vi "Freefield Calibration.vi"(11 "IO Config File":path) -> ()   [LabVIEW 2020]
uses:
  epl-vi-lib/Utility VIs/Conversion VIs/Create Waveform Cluster (2D).vi
  Common VIs/Mic Sensitivity VIs/Cal Mic Sensitivity.vi
  epl-vi-lib/Connection VIs/Type Defs/CM-IO Type.ctl
  epl-vi-lib/Utility VIs/Math VIs/FFT x(t) to dB,Degrees (2D).vi
  Sub VIs/Tosca-Globals.vi
panel:
  in  "MicCalFile":path
  in  "Cal Mic Sens":dbl=-146.12351367888365 caption="Mic Sensitivity \n(dB V/SPL)" format="%.2f"
  in  "Meas Cal.M.Sen.":bool caption="Meas Ref.M.Sen."
  in  "UseMicCal":bool caption="Use mic calibration file?"
  in  "Smooth?":bool
  out "exit signal":bool
  in  "Exit":bool
  out "Abort":bool
  in  "Go":bool
  in  "Mic Gain (dB)":enum16{"0", "10", "20", "30", "40"}(ring)
  in  "Speaker":u16(ring)
  in  "Stimulus":T1={"Min Freq (Hz)"=1000.0, "Max Freq (Hz)"=50000.0, "Freq Step (Hz)"=50.0, "Waveform"=enum."Chirp", "Attenuation (dB)"=30.0, "Sample Rate (Hz)"=100000.0}
  out "Stimulus":cluster{i32, dbl, dbl[]}(graph)={0, 0.01, [-5.268198912753946, 0.15472436668775827, -4.936105719139354, 0.5336653168213406, -4.480102088018833, 1.008248465978206, -3.903407217524864, 1.5781086395910813, -3.213473335937858, 2.237701095068591, -2.422721892763888, 2.9756425911209785, -1.5491700358431084, 3.774205049267688, -0.6168718777938913, 4.609039499746465, 0.34390998389595134, 5.449215840646172, 1.2968922089759771, 6.25766663004243, 2.2004060816056343, 6.992118503588821, 3.008559346676577, 7.6065806282854345, 3.6729832875045987, 8.053433812076703, 4.145191339609901, 8.286124945969407, 4.379529507442163, 8.262418740636797, 4.336639279211482, 7.948093002561976, 3.9872822576766853, 7.320887614931534, 3.3162960756284035, 6.374435881980438, 2.3263695423908826, 5.121827480696606, 1.041250208545094, 3.598385074021946, -0.4920590232314779, 1.8631940827313715, -2.2025827080037574, -0.0010789574010842727, -3.996583101760993, -1.890495716744668, -5.761066652896276, -3.6845867196464788, -7.369807605524503, -5.253642640589705, -8.691888804601312, -6.4684195433316845, -9.602471024635907, -7.211803962263614, -9.995161830161347, -7.39162801642351, -9.794993105247707, -6.953467759606452, -8.970676902555233, -5.891950107327308, -7.544548237759553, -4.2588955339080545, -5.598484435293005, -2.1665998238617026, -3.2741767472418277, 0.2152325190333627, -0.7664729930576428, 2.669906820816478, 1.6908628776126302, 4.951744405784315, 3.846728261111973, 6.810894958294772, 5.460238707232009, 8.022997056956738, 6.331701759997024, 8.420539991290203, 6.333322125748589, 7.921776492633485, 5.435126476754877, 6.552446009009378, 3.7212991072610446, 4.455616406177521, 1.3925580613028812, 1.8858143442848072, -1.248492813884001, -0.8146341545862441, -3.8299221367236385, -3.2565671744760047, -5.958940837626473, -5.058652800945861, -7.28105198504492, -5.908941633849172, -7.541607328468995, -5.62378790744937, -6.63930777826804, -4.193115712222552, -4.660523620731457, -1.8013279613465976, -1.8847202037939093, 1.1842821697169106, 1.245000257577141, 4.260920175874573, 4.186397559561409, 6.87014224603152, 6.390599266533814, 8.499413795406833, 7.408308512375469, 8.78791295611658, 6.9897096713384315, 7.614861791824929, 5.155665436417732, 5.148471552216474, 2.2200736523520286, 1.8384841744623541, -1.2492218903049734, -1.6547038647773231, -4.531415502827719, -4.5875395794318745, -6.9012718876253345, -6.2956683656605055, -7.796639209855521, -6.356893664883222, -6.966612381173948, -4.714378044620799, -4.5603500004007325, -1.7230878322395136, -1.1252562365070526, 1.9034883988795923, 2.497808688702551, 5.246230005199975, 5.368578882073053, 7.4052822320392195, 6.689865512517134, 7.744589066651802, 6.037248961757495, 6.089605211597301, 3.5086613607099446, 2.814876655617855, -0.2603888568289086, -1.2188345294968457, -4.2380841595994045, -4.8785567401632814, -7.271376040922885, -7.077982229264194, -8.426667824565865, -7.1146351776726355, -7.296582121874083, -4.91986703319471, -4.169554633763585, -1.1293660738626015, 0.010491176358083346, 3.0712510234576733, 3.906409710496473, 6.300635894383965, 6.208952288616812, 7.437147684721125, 6.088644097766557, 6.027009247486187, 3.5212689620124986, 2.4930586247443416, -0.6457377872059515, -1.955346718576959, -4.940282413435899, -5.711814843262388, -7.768627179368542, -7.347657247363305, -8.010338407972391, -6.170204268617173, -5.483086055701031, -2.542906791186741, -1.0782044818065517, 2.187214902901886, 3.523630389730563, 6.167577492029727, 6.484585996632547, 7.768138306867664, 6.561596145324061, 6.278028385852266, 3.669742401891252, 2.267554919961306, -1.007135728576333, -2.5775918990285076, -5.454066706038607, -6.130112604803326, -7.670031202620425, -6.74903575803095, -6.575429386402428, -4.059732150963223, -2.566509572230266, 0.7941239410315287, 2.5800169685090917, 5.598533855668952, 6.469880615500485, 8.068262457243836, 7.213875021881164, 6.958454426976153, 4.387760938721065, 2.743633964491285, -0.6698285889953203, -2.5217172717892637, -5.436188670521526, -6.165478739199827, -7.440405214262041, -6.254625534425835, -5.563666428209676, -2.659960840977406, -0.7120378511037083, 2.7734736842514955, 4.561588179801471, 7.124215225716654, 7.371101211272586, 7.95487245705814, 6.091227796135417, 4.7104548555846355, 1.347640330347287, -0.8629413755604299, -4.2223764019046985, -5.6078946806208405, -7.403915239034967, -6.73948774271203, -6.280289141360928, -3.528182677804495, -1.4537578508184592, 2.151691445284337, 4.1924968824838205, 6.841173520638716, 7.163959080313049, 7.5742728334487355, 5.5198442779216625, 3.7800645182637878, 0.1883118086117216, -2.2308126826036725, -5.4902619476836, -6.626836451688596, -7.83306618297459, -6.508973280723542, -5.244810874956672, -1.8952004157835538, 0.606955058514041, 4.151452584017139, 5.7742997100602995, 7.483505877443789, 6.653165701726559, 5.707777580290299, 2.527839497455207, -0.0421815205393363, -3.785098469420861, -5.752805962190212, -7.801424804765037, -7.307010775975443, -6.564461661738033, -3.5029015548473668, -0.8999257692145889, 2.920120961873664, 5.031772146518852, 7.168610599551956, 6.7414300295566925, 5.961794404745086, 2.8441582282215334, 0.1338514074630595, -3.7271586992243555, -5.838810424147609, -7.843217323575976, -7.226392564538584, -6.172779494816889, -2.828986923398876, 0.05150957118887926, 3.898227328017297, 5.845970214987304, 7.487635305665838, 6.438529917848418, 4.922829795746704, 1.2708589242126918, -1.7202877354631272, -5.354532449742658, -6.832245596337666, -7.761997073930687, -5.961194594103097, -3.7683588570341477, 0.2570696544039717, 3.2603785999713053, 6.454848503138453, 7.173169225483685, 7.133981612463877, 4.444211132070024, 1.6238581609609706, -2.5228235439964717, -5.117128911369266, -7.3704847014121615, -6.861442815771931, -5.538160313137008, -1.8790767794661158, 1.3859193207825076, 5.2561678116596635, 6.937544346116766, 7.793213605118417, 5.796759070135655, 3.23732380929227, -1.0067099591150688, -4.056792333319176, -6.867337270546484, -6.926157676049868, -5.9480823057991135, -2.437329342060352, 0.9410718377756682, 5.003300952506423, 6.921678493302532, 7.870442069799751, 5.868846798920639, 3.15138312423561, -1.2262523447841607, -4.360520562115179, -7.039550600472367, -6.8254540193292925, -5.425058430665295, -1.5714782594174603, 1.9871958828743264, 5.860576249209403, 7.278450929372396, 7.435537663444447, 4.646116714214319, 1.3304854578842464, -3.142825361033163, -5.839027496935253, -7.53427953572099, -6.11784564901339, -3.587066735821253, 0.8669398004524809, 4.309913558664775, 7.230064109838996, 7.149607180067794, 5.619711454466257, 1.5585791296402056, -2.232363770655005, -6.085028073428171, -7.244657101692211, -6.844902187954905, -3.4915908929143473, 0.2346856222382626, 4.619909355449498, 6.728626808274241, 7.335598055639178, 4.738791826086019, 1.2546580511285206, -3.434169213629472, -6.294959617165018, -7.811616176072592, -6.006298392634771, -2.9243282833783684, 1.8263339552561098, 5.177408699038257, 7.38622013370554, 6.245568226203343, 3.5497386756087486, -1.18031166283291, -4.877402106803235, -7.624562302507592, -7.035732919059846, -4.691843955635915, -0.03916102015782511, 3.8698153755841718, 6.981994837389917, 6.781956858196558, 4.686291468984885, 0.09779697780872901, -3.9400841946319662, -7.263479231984435, -7.274681327948595, -5.282643435522408, -0.6918479981595833, 3.443619629756007, 6.865576168533289, 6.940338729493144, 4.932275215985484, 0.30236537946239417, -3.8570808228379367, -7.2075454948857605, -7.129379631590378, -4.91267407834013, -0.1361934643380461, 4.040346868467215, 7.216601071667613, 6.845491418147147, 4.32066005828306, -0.5985992815288892, -4.663224734534017, -7.443500502488409, -6.5381869393898775, -3.5301140426186146, 1.58258498272196, 5.4563056048440925, 7.687018074977699, 6.110612696861447, 2.5881403888345274, -2.6005475301936087, -6.04199444453435, -7.444864092474775, -4.992383767520014, -0.9077444233852652, 4.2342698830343375, 7.01788981780445, 7.387987352809551, 3.9967242643582868, -0.5092571824830199, -5.296631172179451, -7.070340682960906, -6.169613293871741, -1.8315435704147096, 2.8599819372393345, 6.919670453017385, 7.356344103481067, 5.080350143682289, -0.007085816050160075, -4.450717216127243, -7.306527333021936, -6.120738321455922, -2.5359997753017236, 2.8835512421863796, 6.487973207603957, 7.654891895746284, 4.7174230342389265, 0.1407496746273733, -4.979227860208258, -7.101779182600751, -6.264092701195794, -1.786090165267261, 3.0961184280731273, 7.05481129330459, 7.071743958604985, 4.167477970081142, -1.2938716831393164, -5.564824614463605, -7.554455584640754, -5.215261753753379, -0.7438685150851565, 4.63733729895058, 7.164584661085231, 6.552007283319558, 2.0676934427885048, -2.992900235336533, -7.04026615832861, -6.966438541255768, -3.7982072924186374, 1.8236464798201761, 5.960125196888981, 7.4140371618339165, 4.405395111049246, -0.5115316522716058, -5.715512079470977, -7.4486956056584654, -5.741118978332028, -0.5258040735298557, 4.421353351307599, 7.372267358024189, 5.741658380261856, 1.3522526983977523, -4.354569651532247, -7.288094350203355, -6.756543775969935, -2.0945874938808453, 3.1769460410787715, 7.042773160858427, 6.387686433421049, 2.4864168062370635, -3.39222429739403, -6.990987053298005, -7.159506000295234, -2.865999786873386, 2.533024409042783, 6.835427877890322, 6.6388697676783535, 2.9382852847908305, -3.017674445230749, -6.8505663481906875, -7.180577760890124, -2.9022704881692176, 2.5923158052172033, 6.925831567928834, 6.631494888469215, 2.7413917763985367, -3.2880358394581983, -6.953415262515216, -6.879496083870497, -2.2247260026423192, 3.3411092530878466, 7.273357193605295, 6.300652326252434, 1.852866676186904, -4.171172991169453, -7.186624607668294, -6.12902354187548, -0.7981910785525986, 4.652176578794313, 7.621054032499265, 5.397615158172362, 0.19659281853413826, -5.495756604067253, -7.219068212498481, -4.655291634956677, 1.3809179893349508, 6.2030315392201345, 7.485967672803411, 3.5807494650504568, -2.185222607280925, -6.832618016206194, -6.503842738222435, -2.1772446291201564, 4.089508811229626, 7.360481851909367, 6.2214480183612055, 0.6382302519063133, -4.886374544928762, -7.399486655729083, -4.4192288260547645, 1.2938205688827986, 6.6250384668429705, 7.171081058582159, 3.2897988000769116, -3.125494623688734, -6.911732715531365, -6.184970877676735, -0.6871977715566325, 5.026819820197494, 7.696981254517481, 4.695321242939161, -1.1624644088507237, -6.4866533422822386, -6.778679367154203, -2.537592715186285, 3.947887510720634, 7.320559752380773, 5.854035586827115, -0.13701600509322034, -5.637873695952034, -7.371155360792105, -3.359976713972514, 2.783840541352301, 7.262662307713002, 6.073547272708852, 0.7547535754815095, -5.477309421766594, -7.320704143407568, -4.076948523339965, 2.53079043139377, 6.879028855078228, 6.360929921143857, 0.6631898541259118, -5.2607397717088595, -7.593198682858205, -3.8811303142164526, 2.396208473538858, 7.097824106814894, 5.938217739780265, 0.438071984502258, -5.827153971326262, -7.3522200770230395, -3.583193416309296, 3.2037473262277665, 7.058746580825766, 5.5798006821120625, -0.7322933754485541, -6.2736137709411866, -7.282641773699037, -2.306637740796302, 4.079753813280838, 7.397921500073831, 4.346996330085451, -2.0204892667542436, -7.193316057455906, -6.356667865026697, -0.7775157490101203, 5.630597151405401, 7.024916096379502, 2.8515434851487265, -4.080310479287762, -7.455819131696737, -5.061730364173382, 1.7409273182319849, 6.716616268130217, 6.300852344279075, 0.23552513221494614, -5.812510898885256, -7.325656715369917, -2.416499935912286, 4.20595340691375, 7.503936045716031, 4.083013830130799, -2.576841185023463, -7.339719634050704, -5.523473316178671, 0.772215866457928, 6.689504274117393, 6.536788709293754, 0.9905473222769816, -5.6786287807560125, -7.072919350903344, -2.492595360069329, 4.610518393169291, 7.431512510272139, 4.008126798735533, -3.1803291782074385, -7.196110375032134, -4.972210543995063, 2.066365564079555, 7.08401321285749, 6.089340041167519, -0.5678580698696746, -6.342892846151588, -6.505666330592822, -0.35841099199108073, 5.985318681299599, 7.233767406971928, 1.7044686545440948, -5.014020375571299, -7.227374527708142, -2.3546475482644085, 4.592417575438715, 7.651973956236934, 3.443675179802632, -3.613300291172199, -7.397790861690395, -3.833752276459987, 3.238215867956934, 7.618538599317088, 4.637769723342312, -2.4043543328002115, -7.284534656947072, -4.8366282120338795, 2.124658179220868, 7.3833563562803715, 5.365786075012751, -1.5286689107614526, -7.101549908881539, -5.4522850675471135, 1.3553539065710465, 7.133510118326032, 5.727854230955125, -1.045904310760646, -6.989677300898881, -5.762167063662348, 0.9757983264882566, 6.985265407399975, 5.801261118091874, -0.9720815649171468, -7.0177242645731095, -5.809234307611887, 1.0039792584619325, 6.987323157037585, 5.6178467367115505, -1.3040770033795295, -7.18811195441027, -5.585445385131738, 1.4444012666063888, 7.123281681225336, 5.156842693841554, -2.026307886941771, -7.438605045603327, -5.032956777454607, 2.2836619932422635, 7.308768914377469, 4.350881349278516, -3.0988289576015937, -7.638971012985208, -4.059037989768774, 3.468094227327584, 7.38592769485375, 3.1079006313030444, -4.428347604106914, -7.588690184326886, -2.5693342094283067, 4.867003222988194, 7.12533243326591, 1.3551207959485267, -5.828292247585097, -7.029386568246263, -0.5255949468199037, 6.231850405988089, 6.252650257500143, -0.8903534092909058, -6.983645855777526, -5.691895386890709, 1.9717723677392618, 7.17394815534516, 4.5211080961372945, -3.4309862355822447, -7.450644081357213, -3.3973230722522314, 4.593486647599771, 7.1980976900131814, 1.8432618772903955, -5.809370417025735, -6.734255164992385, -0.21420006265580677, 6.731007664855428, 5.836152549849441, -1.5342489824366763, -7.304934828415726, -4.481433783316572, 3.370137858915535, 7.566115459500614, 2.901650517094279, -4.887209306299948, -7.0955274440845155, -0.7812482646532353, 6.373774279295743, 6.3445202532922576, -1.1890072905137836, -7.0452332506031565, -4.644004854227093, 3.541947226113793, 7.505870972955428, 2.8632692659772947, -5.211202610046928, -6.763474275312138, -0.24006791276950218, 6.890503265856279, 5.7417500312555525, -2.0055534494094984, -7.33737276359952, -3.4769048139735705, 4.604716101023941, 7.4088764134763965, 1.1882987138543064, -6.177258620815541, -5.986828798179214, 1.8531483144550864, 7.412557985728574, 4.13192051037388, -4.269852095724912, -7.1065896117768474, -1.1471485015074143, 6.512186887113054, 6.0211927787580235, -1.742035149083485, -7.375702831608887, -3.5159499563671814, 4.708021360701314, 7.21681111293023, 0.5253731768581403, -6.637719013896884, -5.472203173475872, 2.835983027958118, 7.4174703354896625, 2.674619443930915, -5.630851885441911, -6.575749936156022, 0.7909319027737999, 7.254060445787437, 4.1722214947775775, -4.2266678223662115, -7.330160415722715, -0.8252888610020537, 6.553516610912413, 5.418876561967503, -3.039107659742079, -7.480630271961402, -2.3188358948188736, 5.917107002494558, 6.084259196613284, -1.8109874183634276, -7.570939769222146, -3.2782185847135095, 5.113155616671117, 6.647524150125307, -1.0022706256615814, -7.349780692491279, -4.103765116699421, 4.629395585382437, 6.821925602548551, -0.2703686909901486, -7.292107730028471, -4.456559373064684, 4.1617649608314515, 7.049200144935046, 0.006196751679581222, -7.098805407130077, -4.731715940350453, 4.108203743544292, 7.013235776847501, 0.18415732468433557, -7.161584281268779, -4.591033378380794, 4.126429376001207, 7.0791935320889445, -0.08855841191627135, -7.135214960218198, -4.380778864995472, 4.553006058302461, 6.883801926906562, -0.4722410686728798, -7.332725197110119, -3.7437692063795662, 5.020095243935368, 6.71171645322024, -1.2985962708294916, -7.3622106844365875, -2.9800400656221955, 5.797291864656931, 6.158816331213153, -2.224937194593592, -7.452801625687471, -1.7381023125659305, 6.468183227507671, 5.449800363739938, -3.518314665836994, -7.161835192560194, -0.32239852080531084, 7.202750217326174, 4.182349566323476, -4.767726810954141, -6.645762480602695, 1.5338234973032108, 7.507271290643875, 2.5982763353206244, -6.100556932988706, -5.456445557052954, 3.415468302893055, 7.451267688369972, 0.4173032991800682, -6.974243481539636, -3.7796132692587077, 5.386226011801764, 6.521837729952901, -1.9391425150286377, -7.362910965180193, -1.3353108448939035, 6.824424409945794, 4.839741670112702, -4.4501670956283705, -6.67827190354844, 1.4212313376951484, 7.578245200127353, 2.137799252458786, -6.378976706181101, -4.977491033689597, 4.343053947340082, 6.968781033772617, -1.0532636822086119, -7.411520461688359, -2.0333166452809386, 6.533476295718684, 5.010056713625797, -4.394771409814594, -6.766415880577115, 1.490592054440969, 7.494701529741184, 1.584510348167756, -6.765875003379135, -4.453721736990209, 4.994836541078157, 6.380014914243036, -2.401240444331501, -7.468034788581953, -0.5629989372293054, 7.1014838380930385, 3.315790659763432, -5.984972866410088, -5.666022464878779, 3.6364444725496945, 6.979129540023752, -1.2187945093177486, -7.520358777665627, -1.7810364268856296, 6.768011954431605, 4.010298267709568, -5.43908213200435, -6.199981869315344, 3.1150740281930926, 7.045375361245859, -0.7962947891099998, -7.579039481647398, -1.9406637419191988, 6.663438416961239, 4.03793806415907, -5.577393444155123, -6.025675155876606, 3.3524447442922387, 6.972745469273113, -1.3615484849416026, -7.54283528682556, -1.2527409352797423, 7.027594011265683, 3.19902479985998, -6.164911155250056, -5.277446467439849, 4.483910180531211, 6.416848405230189, -2.6831794233556474, -7.371094897377518, 0.499084165392108, 7.363843648896164, 1.5304658331085685, -7.066614597985621, -3.4987236286655747, 6.012514092209379, 5.1208152069279045, -4.726888892085679, -6.339980396690471, 3.0280610687405236, 7.170596716367043, -1.2304909909162949, -7.405376290549076, -0.6024544481206826, 7.35908916056172, 2.4111240157942073, -6.661273890158799, -3.9276309786496135, 5.894783285661235, 5.359498291875047, -4.51463386051595, -6.269245318061246, 3.3201813644649016, 7.112088310331547, -1.5931758561482559, -7.31157058232791, 0.29015178357394994, 7.525804393455864, 1.460715386346605, -7.070159289724406, -2.6057496859138713, 6.7447285383244, 4.1321168455714385, -5.791908477270606, -4.946633731136702, 5.085574659161792, 6.099100503146692, -3.8367309287034863, -6.511230043001646, 2.924531690254378, 7.234452167248464, -1.57584944954651, -7.256400220654791, 0.6111775712249089, 7.5673672000412555, 0.6766388457356355, -7.268044098909321, -1.581971016051082, 7.22885018125015, 2.6970731358613524, -6.705531672246968, -3.4775791751495437, 6.398472526999905, 4.357344965207453, -5.753451680296769, -4.988423451542873, 5.262443474031636, 5.611980042519988, -4.587086048407322, -6.099349682927693, 3.986351788380044, 6.47678241551341, -3.3524691857209836, -6.844753534998459, 2.701548116804122, 7.006193817072543, -2.158652789159005, -7.287278289511652, 1.5019584261002876, 7.273655545638933, -1.0785289881197602, -7.500700710838877, 0.44759570639718305, 7.356818396055228, -0.1546115414097622, -7.55789351243099, -0.42850824296939377, 7.327754353537282, 0.5931062701371723, -7.523447506788368, -1.1123666046166072, 7.247374449411044, 1.159185250634697, -7.449901616205839, -1.601621464253939, 7.162883318038112, 1.5458102912476162, -7.376367409426471, -1.899450820362437, 7.107098850147537, 1.757433193486522, -7.328452716552958, -2.01011509029858, 7.098661566725419, 1.7971510342778039, -7.318639128727494, -1.9361943763208442, 7.142434753368789, 1.6648073852202323, -7.34656075225719, -1.6774727637188105, 7.229689176548243, 1.356767167247066, -7.3989251846347255, -1.2314375310024652, 7.337952987361621, 0.8673536650984877, -7.449104232450871, -0.5954147670466945, 7.430690391118509, 0.19198443473597804, -7.456709150233372, 0.22960505823745772, 7.457261141055401, -0.6679619947529072, -7.367759400114487, 1.233451712394734, 7.353906046052044, -1.6986391934598437, -7.116342517234951, 2.3897741199596085, 7.0467730089811695, -2.865978782777268, -6.628896894855508, 3.6481691703374213, 6.458171005742338, -4.107611838917467, -5.832329492619806, 4.926704590233439, 5.517187548057526, -5.326147906215478, -4.666950020678309, 6.1069514253257315, 4.175347079673148, -6.386398813093694, -3.1044632212483703, 7.034546908113638, 2.4269197401967855, -7.1199582301857305, -1.1698218514798955, 7.5289510859962805, 0.33166218770904743, -7.340876726227963, 1.036471629569474, 7.405929210953934, -1.9647783612357537, -6.875407655143098, 3.321820293891651, 6.5147262079528465, -4.220434647492109, -5.606263402883918, 5.399664376298967, 4.788269349404898, -6.106439584183898, -3.5270227628406747, 6.912582638807577, 2.2988016760946346, -7.246217682554448, -0.7954174368579265, 7.488884339759199, -0.696205046129878, -7.290279059088492, 2.2334387254592376, 6.8343818182803435, -3.7400204302108024, -6.022587668123615, 5.018196863144114, 4.848106750641775, -6.21925088014328, -3.478780042622402, 6.909607072125957, 1.7330235675491468, -7.480914404048713, -0.038068175043771364, 7.305467184454901, -1.9445184173264187, -7.021243676354168, 3.563101460592977, 5.863706867127409, -5.30019256611829, -4.709091588781449, 6.345380550046475, 2.716281625948426, -7.320885780942076, -0.9668260764181981, 7.349045869067955, -1.4098828132495977, -7.190992713412808, 3.195376456475068, 6.003887408701125, -5.2694991187727975, -4.67572044811709, 6.383900715158481, 2.485755581766223, -7.437021874893461, -0.4039453612946393, 7.283973152152595, -2.1241094084617758, -6.86536613448874, 4.142265082449705, 5.267387667723275, -6.0546740711016405, -3.4768414745568266, 7.064626570553517, 0.8872129934270778, -7.492742844867697, 1.5237077317000276, 6.864034305240107, -4.069849674206927, -5.488323475199265, 5.917276189626665, 3.3271072713237677, -7.197653739918008, -0.6908421330394027, 7.408965533095865, -2.025187400995709, -6.654673412230403, 4.612716930967556, 4.923420046978757, -6.392242558651788, -2.3878636424510074, 7.464374614775881, -0.4523468148347535, -7.107263295567351, 3.4119278069323333, 5.939846181696391, -5.663739538586874, -3.392413997277974, 7.23495552715241, 0.6557471437831315, -7.304522630414506, 2.695122036717736, 6.382835657680963, -5.113094128823615, -3.9498736502053196, 7.1336670310335295, 1.0930032543939112, -7.283955770137286, 2.37658627156351, 6.558282885289726, -5.049018440869571, -3.9488754943513236, 7.094554010811722, 1.0430377448665433, -7.318649642280466, 2.6642916523307383, 6.318810357585746, -5.3080138447779435, -3.5879739009830725, 7.304902607746897, 0.3105868538709081, -7.173051569327158, 3.3416830891067137, 5.800843030737964, -6.016406429204358, -2.6099276973106673, 7.437985995874678, -0.8968525383556791, -6.885618752640273, 4.533134164207345, 4.650562518060876, -6.770810693679945, -1.1458164399628608, 7.4553189773982576, -2.730496942614673, -5.968048217614874, 5.8160937074042485, 2.9176196034845336, -7.445941801944742, 1.0423410434064015, 6.761704783590702, -4.743195289910076, -4.343459165795438, 7.023307372493463, 0.29477931334295804, -7.30412375074616, 3.5280082327773696, 5.181401901962682, -6.6884161105715005, -1.5924568517472815, 7.301053959440679, -2.7713986307337652, -6.022404331580274, 6.005444758334429, 2.2165403487578135, -7.537010365189257, 1.8386853210947882, 6.1943032816067305, -5.8514795104740305, -2.991137106537487, 7.263806422763899, -1.6325202796756646, -6.647602385093664, 5.378321463779326, 3.009420866089287, -7.480091922619858, 1.2201284744109158, 6.467236472992606, -5.573021530453243, -3.238750984296706, 7.2626510188566336, -1.5472406664052007, -6.594104792863606, 5.526892945820245, 2.784430587244071, -7.477451135507415, 1.764318217766512, 6.193312632869459, -6.005931672119629, -2.385004143128125, 7.371659778348825, -2.5316991839326146, -5.851015812061519, 6.3777597681171905, 1.4848907989979554, -7.359259216876276, 3.383746118747219, 5.121608727602291, -6.8870327556741024, -0.3419386359895471, 7.122433920514759, -4.4142022511899, -4.030839287920141, 7.372883921446936, -1.0104055374690604, -6.453195007736038, 5.652879886395455, 2.7192391185379594, -7.414473281753894, 2.822296941112396, 5.587859533857973, -6.505030504056118, -0.6982352824551419, 7.3427523387040825, -4.375716527149005, -3.797948598192084, 7.403901054754664, -1.2467079300186006, -6.206915079577845, 6.219994502035965, 1.8812855918849696, -7.21356980341845, 3.7976300394487357, 4.768156324999836, -7.090085790515599, 0.9925870731971558, 6.620623009652825, -5.632886555814452, -2.037184094810564, 7.575272088198509, -3.5305398861309003, -4.476744989356374, 7.240062304831142, -0.8131785901705556, -6.383254786545178, 6.133344940765426, 1.7437276038378704, -7.2172822408269335, 4.1293447739209785, 4.184032033228714, -7.3455305194741225, 1.916008769188193, 5.880822464727152, -6.4792053898117565, -0.5970589961541429, 7.094065192957407, -5.187917469318833, -2.757153061838549, 7.396113436351452, -3.2854972826184152, -4.772191206712707, 7.240321435536306, -1.390723203248624, -6.116260305539997, 6.326525799026532, 0.7144743302731418, -7.149271494643727, 5.205911455748185, 2.4630009343718093, -7.461037971557037, 3.606922021743368, 4.167991786044972, -7.522291187896895, 2.091294519815033, 5.341956985845469, -6.98166385006456, 0.34819064048930004, 6.393126140437912, -6.360560920695885, -1.0955731847071088, 6.894051332299561, -5.31128869421998, -2.6148139354445465, 7.3176903788025305, -4.361174242102421, -3.7248310077122744, 7.262144728895676, -3.1334741187855837, -4.859125077652972, 7.232020831764564, -2.140904686041697, -5.561579941593053, 6.82217355800608, -0.9673442783996639, -6.307003775872721, 6.546333483332153, -0.10889010405423968, -6.649335246347242, 5.979804185381586, 0.8864521852085172, -7.087513362547955, 5.63525805083038, 1.5319780041595186, -7.17053248948962, 5.063007834971533, 2.3068148074477537, -7.409581717960173, 4.773225847086141, 2.7243202913087545, -7.339554481284766, 4.292218234970269, 3.2821597294340616, -7.4775878501999715, 4.130472963240131, 3.4859959755485463, -7.34012884129945, 3.793660480785639, 3.8458047177268, -7.44779328506394, 3.7963055342514855, 3.8544734570010535, -7.2970421897086934, 3.6265937914663144, 4.030757146799401, -7.411385874473106, 3.8058030970737717, 3.8522276659686474, -7.266874913102797, 3.806246091744156, 3.845238144087636, -7.389895721484403, 4.156818465616575, 3.4716794649841134, -7.235888055513042, 4.3135530577508225, 3.2664169443963242, -7.334222845400351, 4.811793140792276, 2.677396155101437, -7.119772494562921, 5.088949016008644, 2.251128502265069, -7.125606361762035, 5.683972067609279, 1.4257376939212443, -6.767245399921996, 6.012080776288262, 0.7650925939860065, -6.584130569254961, 6.6124766289028, -0.2957169615208086, -5.976538959742762, 6.875099697236678, -1.1671936162978764, -5.496883472445029, 7.337906727964457, -2.408418255116013, -4.539207794871777, 7.366080415601138, -3.394921421033718, -3.6811574912810503, 7.5005479621525435, -4.671748894791566, -2.3254495527029784, 7.090252623782934, -5.5733321909020255, -1.0925326475946708, 6.693542404862393, -6.62916932518457, 0.5878143467857476, 5.663594405868356, -7.1374088657337555, 2.034690139061274, 4.603217845992474, -7.626149145285267, 3.7780707617726983, 2.901644568189083, -7.382220854118887, 5.07131765514263, 1.2406343061383283, -6.969894247839067, 6.412049108213185, -0.9225769167783797, -5.713714378933332, 7.012943400617945, -2.8037500151205674, -4.272202999499362, 7.385704926316464, -4.871283360284997, -2.0677727581517775, 6.770669893032357, -6.257354174975097, 0.09388756265418087, 5.781674164983426, -7.408537555470525, 2.6607714855204208, 3.7854099254741804, -7.4632547405994085, 4.683998588640356, 1.5930505968580824, -6.972103264862576, 6.536723624612685, -1.23234583482215, -5.229875124110247, 7.241220620442128, -3.661784658335817, -3.044333861500277, 7.2701217022324265, -5.990169988709713, 0.010601058375152657, 5.83530790274474, -7.116313518357464, 2.8167495544053627, 3.7391157119716016, -7.432194251015661, 5.5774787332529066, 0.5736924884437822, -6.073795748434888, 7.056885013617561, -2.438869392571146, -3.859268385910383, 7.566825583605902, -5.397328715537654, -0.4315930839781542, 6.1855017982488025, -6.92993031010169, 2.8468492299796297, 3.7847227402904178, -7.291276430888082, 5.945921857850861, 0.1068066140819823, -5.5527130408794045, 7.361544561252553, -3.302854764414877, -2.713782604756743, 7.335432635857689, -6.272811942495798, 1.3077181212058375, 5.014901385184877, -7.204035331726785, 4.735019252899437, 1.6295085128878233, -6.420071110229997, 7.268196155607813, -2.645237058479404, -3.277007289895888, 7.304098779984496, -5.783672176568736, 0.6385538744153036, 5.406018520513537, -7.439435296959046, 4.835105570456163, 1.3124691389736631, -6.1836952557524585, 7.1011206267826745, -2.921447554485646, -3.042899043677755, 7.24305407094255, -6.51929379287791, 1.692989251741919, 4.288379249143579, -7.291352432686731, 5.493894263830298, -0.025555092643484087, -5.535061544588668, 7.51995648018632, -4.791451749474087, -1.0620161154010102, 6.013119972602393, -7.220192135671134, 3.5503435214875694, 2.1990106921883044, -6.884413948062836, 6.995941269328584, -3.1051878782565536, -3.0054815612269277, 6.788886138600794, -6.680281702352021, 1.9447621049865997, 3.6074132631046685, -7.465930601719045, 6.332135569697447, -1.902140956931149, -4.122664682247093, 7.0474697348311865, -6.182225617763155, 0.987450504016817, 4.307318187590881, -7.646712207746921, 5.94143549484391, -1.3449584990348453, -4.528858050616823, 7.10768785408077, -5.99784833818804, 0.7794946356385093, 4.42108425287248, -7.6375498884863315, 6.00203369972859, -1.4728095957933145, -4.296858306756864, 7.085913464756461, -6.203031539261085, 1.3332641517130461, 3.9667943343253453, -7.4504035593841635, 6.494700043196976, -2.2817930240452595, -3.393648821480432, 6.877443616438691, -6.698712303866614, 2.602286685842846, 2.8427906367481475, -6.896652714707194, 7.199266294726993, -3.7025533769798784, -1.7105730842705416, 6.17286490673505, -7.181228790818576, 4.411974362603514, 0.9111133126008619, -5.623338683285598, 7.655856904023626, -5.481327278263599, 0.8038624431073437, 4.539746330470848, -7.1028272275444815, 6.3144195946827955, -1.8034793181298114, -3.2483904158245327, 7.167792474870116, -7.016022070941451, 3.8957151466123237, 1.649844329305818, -5.7393904447400015, 7.4591403195870685, -4.814300882898643, 0.32087271721727045, 4.996538698910781, -7.2978703082598315, 6.711130057911584, -2.293421830197837, -2.5369531029189907, 6.693858365069438, -6.932942720410846, 4.400709250099052, 0.9019034938261111, -5.232011317335216, 7.728515412451815, -6.070763570839876, 2.185089788906171, 3.18497512246112, -6.485072255501045, 7.19882653714837, -4.060491616072468, -0.5652155517907376, 5.395678763147044, -7.445899300511558, 6.5232258101982925, -2.408875508855543, -2.4414291294209893, 6.3649006703149045, -7.177372308663665, 4.902131545975449, -0.27653122193389595, -4.440752073311796, 7.311123039342662, -7.0466075550413985, 3.748393713743228, 1.02259006190719, -5.4001375456527505, 7.232087194276419, -6.112028514800706, 2.095552535628311, 2.5832017567243586, -6.5448710518470605, 7.464729024695672, -5.721191514224175, 1.2430983905085926, 3.2196486214937696, -6.775658303016905, 6.966918995244128, -4.802347606366615, 0.056554421507401656, 4.166056710700625, -7.386812543479487, 7.064953041110443, -4.6480399347448955, -0.21922722215183704, 4.242266849206085, -7.224540473962878, 6.609292906955443, -4.069812515834563, -0.8140872189924999, 4.723683236382706, -7.581082223109541, 6.8943465836242614, -4.3427985603489425, -0.469462178283496, 4.364039955886553, -7.207588595028469, 6.660750006909448, -4.1956857038108595, -0.4647348677075911, 4.44014636783252, -7.378388720535737, 7.177959419666832, -4.910104882295666, 0.4978317402166672, 3.62107740135188, -6.742755836737935, 7.07716617306676, -5.133176897284266, 1.086507371731375, 3.1923705588144142, -6.5627663115627115, 7.601303168125049, -6.137992714004316, 2.6142504029866966, 1.7653083915202596, -5.3995497165282895, 7.265693650955702, -6.455623108589378, 3.6457992451237335, 0.6913697570813713, -4.540701657216105, 7.2941918125858995, -7.314651755628377, 5.443451838379087, -1.3929159782414229, -2.5253539878920357, 6.117504128857631, -7.103452803831995, 6.39270593621441, -2.9556306733107145, -0.7801763344754337, 5.025576518112384, -7.025156450689789, 7.653611065280121, -5.212964074433305, 2.0237385995352533, 2.514655796524144, -5.416700313688903, 7.437789037496328, -6.35146670518208, 4.137993946935715, 0.16865462993144453, -3.659568612997817, 6.927332596263885, -7.431917921081369, 6.612557912757376, -3.1852214785674757, -0.3530387039328028, 4.441250109869715, -6.515927788053014, 7.352441731410537, -5.44245088809795, 2.558701451575206, 1.6384412548980578, -4.909561009186394, 7.3571682926497814, -7.413776024981069, 5.903184192786667, -2.518499192366596, -1.185233442622366, 4.752469608436264, -6.805773431696228, 7.147484134991613, -5.476729606965427, 2.3647584242330506, 1.382949174298675, -4.8930453362168285, 7.065405272198576, -7.672280695037907, 6.153253878954251, -3.436302020902229, -0.4226128698540964, 3.7180407541296425, -6.480348766354185, 7.098179399949354, -6.474136454485295, 3.6426532951535378, -0.5222610682769486, -3.4399270792713987, 5.910215565733283, -7.777677166092991, 7.077816746051623, -5.594645433613681, 2.02223732342793, 1.0837745270214958, -4.775851271391948, 6.404313630179907, -7.457579802725881, 5.8363753036487855, -3.8172154357841546, -0.052325203982481555, 2.9882568383629526, -6.268888647828698, 7.2689154904253535, -7.686975230614976, 5.566010612822198, -3.228507996011473, -0.6363758037337859, 3.4308357711670774, -6.297269204086456, 6.975500085117721, -6.945698825894605, 4.69016617948911, -2.1460494539852277, -1.5417150317653114, 4.332408838518213, -6.8705231353602745, 7.557807273249924, -7.270805211030309, 5.188932445833566, -2.511446883467661, -0.8982089125610887, 3.8346601306280266, -6.163622442033808, 7.151556709854065, -6.798471493733942, 5.138369404823166, -2.4099118004303173, -0.6616980407435415, 3.8512448844467184, -6.108996369005021, 7.6340437522303395, -7.437771191224908, 6.421084881867248, -3.8022520400649107, 1.1474518489641143, 2.286587898785318, -4.578856429007744, 6.775340417057683, -6.971198708068286, 6.78505682712836, -4.52806759715431, 2.4105029477573092, 1.112481056787596, -3.4785918328681715, 6.351874561908106, -7.164147298952606, 7.959530077199515, -6.414124870856378, 5.034131310812939, -1.7691310832533527, -0.564047032536154, 3.9150164777187664, -5.453627230322887, 7.266337798570007, -6.788733230111092, 6.384115717306525, -3.8763587734437794, 1.8557407551913272, 1.5363012529118347, -3.6991024316185057, 6.363363399649101, -7.1876391635132855, 7.951182638424688, -6.761792831703346, 5.498582338374045, -2.750840348462315, 0.39029592983396066, 2.6262177119682213, -4.645865154596283, 6.519173521741171, -7.023548538732575, 6.946115491778043, -5.60984411368266, 3.75066742179143, -1.2162056218274702, -1.4178741499303906, 3.907530046503666, -6.01021423028047, 7.24503209243035, -7.85464809147212, 7.23111879607223, -6.165309620886804, 3.934962021362205, -1.8309267127370736, -1.063152858114128, 3.086975435248174, -5.475044135932798, 6.349672450482585, -7.3667386358493205, 6.54289328234181, -5.986677586550185, 3.6446452653741734, -2.020782000511449, -1.0466393445324098, 2.7829432157407172, -5.53525515857639, 6.405254099349906, -7.992905660269564, 7.397545241785114, -7.489087683170065, 5.4288857102026835, -4.306391039205678, 1.3481236453529608, 0.24456578057710482, -3.2173567916128936, 4.39135943096623, -6.528046221926871, 6.595337300485438, -7.3873494827883155, 6.10449021213772, -5.544248846760801, 3.1751534276434694, -1.722366457239506, -1.0843826809067085, 2.6978090978033453, -5.155494661255595, 6.197820180898688, -7.654662704144305, 7.643250594322533, -7.78725152771682, 6.633309993865312, -5.568244075889204, 3.580785530238637, -1.7622350662739208, -0.4752522546902493, 2.40866919524754, -4.236566233671953, 5.673014156944682, -6.559799236743594, 7.09665122804632, -6.786760078597537, 6.334110060962726, -4.9019201672270345, 3.6855866076011115, -1.4903134691589983, -0.035339203799032035, 2.469952832491278, -3.7647855622532918, 5.9041092243934035, -6.495071508526586, 7.935051201114419, -7.5369280417086815, 8.097232275909386, -6.673282892314059, 6.4236050163663325, -4.177563813006, 3.3983254502663707, -0.7079091459078674, -0.19700483897050605, 2.881752542441214, -3.4932084715589706, 5.758091883852156, -5.74259463340116, 7.297820081354564, -6.478547105850378, 7.209839208206819, -5.595422628049647, 5.571009356183328, -3.341000721607474, 2.778598391041956, -0.23425715478056194, -0.5597031380088721, 3.0644702027601585, -3.7670492512600147, 5.897820652995271, -6.236972852878438, 7.739157488663354, -7.543547188170974, 8.280732591336193, -7.504650496720316, 7.470644612084793, -6.192679953662271, 5.498650578141172, -3.897955422581154, 2.7405024745573643, -1.0580135805474216, -0.3234505793249378, 1.829941671555072, -3.1975876455216596, 4.295992277660061, -5.451988004088022, 5.969393781338585, -6.782887910930249, 6.625875179664726, -7.045910611220712, 6.206473719659867, -6.26091611224869, 4.809253398866243, -4.5920111312568, 2.659266657499252, -2.3094855058906987, 0.06450620946791424, 0.25801896386818457, -2.633684476159889, 2.772835758538232, -5.107976541452407, 4.932091456014839, -7.084143784987004, 6.501046364397496, -8.36806390979394, 7.333326855209402, -8.8591505270234, 7.377646525308829, -8.55078907516914, 6.672438728293716, -7.519903948601991, 5.331080627898659, -5.908734720274895, 3.5210350437129154, -3.902254766858653, 1.4403238815014463, -1.7045150121628725, -0.7056072539422032, 0.4833248828667927, -2.7242219290307896, 2.481253855807945, -4.451804397732298, 4.143744964845767, -5.7641366321582455, 5.367731427325334, -6.581846951995106, 6.095435319977688, -6.870905400088031, 6.312742146377243, -6.6391307889492, 6.044112974706465, -5.929784574261516, 5.345153089878375, -4.813378185576395, 4.29394027247128, -3.3787467178763175, 2.9820939551746326, -1.7242817751942958, 1.5063777026278393, 0.04999215840351548, -0.038592247188749935, 1.8490369770110349, -1.566180502704833, 3.5878677172503783, -3.001956329097272, 5.195002769454339, -4.286321452431311, 6.614378769667364, -5.3756797669265355, 7.80591442773415, -6.242369039243872, 8.74496988413574, -6.873618389291001, 9.420974896985152, -7.269806725470315, 9.835497254611841, -7.4422839283846205, 10.0, -7.410986098531348, 9.933499797995244, -7.202035688424697, 9.66029563928829, -6.84547280591735, 9.207892374793566, -6.373220050168512, 8.605201258042488, -5.8173432099340925, 7.881062366060826, -5.208636048832144, 7.063102929999032, -4.57553019921288, 6.176921747554907, -3.9433110346834335, 5.24557277245882, -3.3336068503970155, 4.289310003143563, -2.7641109338379293, 3.3255499629309044, -2.2484931464836535, 2.369006298505884, -1.7964583939632761, 1.4319522464482368, -1.4139128212047907, 0.5245699414692682, -1.1032038220195375, -0.3446500832260673, -0.8634062356042506, -1.1684910062417149, -0.6906338046178808, -1.940600436571016, -0.5783616248202543, -2.655112322318282, -0.517751584541918, -3.3063188039851843, -0.49797843339505965, -3.888407596704841, -0.5065589657816423, -4.395277932282514, -0.5296907331436173, -4.820446023285823, -0.55260960786453, -5.157049223297509, -0.5599773115618993, -5.39795628927423, -0.5363105805493877, -5.535989103840361, -0.46646284424612283, -5.564258565776937, -0.3361669974163001, -5.476613783627737, -0.1326439116728561]}
  in  "Averages":i32=128
  in  "Stop":bool
  in  "Show all":bool
  in  "Load":bool
  in  "Clear":bool
  out "Path":path
  out "Acquired":i32
  out "ASTF phase":cluster{"Frequency":dbl[], "Frequency":dbl[]}[](graph)
  out "ASTF mag":cluster{"Frequency":dbl[], "Frequency":dbl[]}[](graph)
  out "Mic phase graph":cluster{"offset":dbl, "dx":dbl, "Y":dbl[][]}(graph)
  out "Mic mag graph":cluster{"offset":dbl, "dx":dbl, "Y":dbl[][]}(graph)
  out "Mic signals":cluster{"offset":dbl, "dx":dbl, "Y":dbl[][]}(graph)
  # "Raw Data"
  # "Acoustic System Transfer Function"
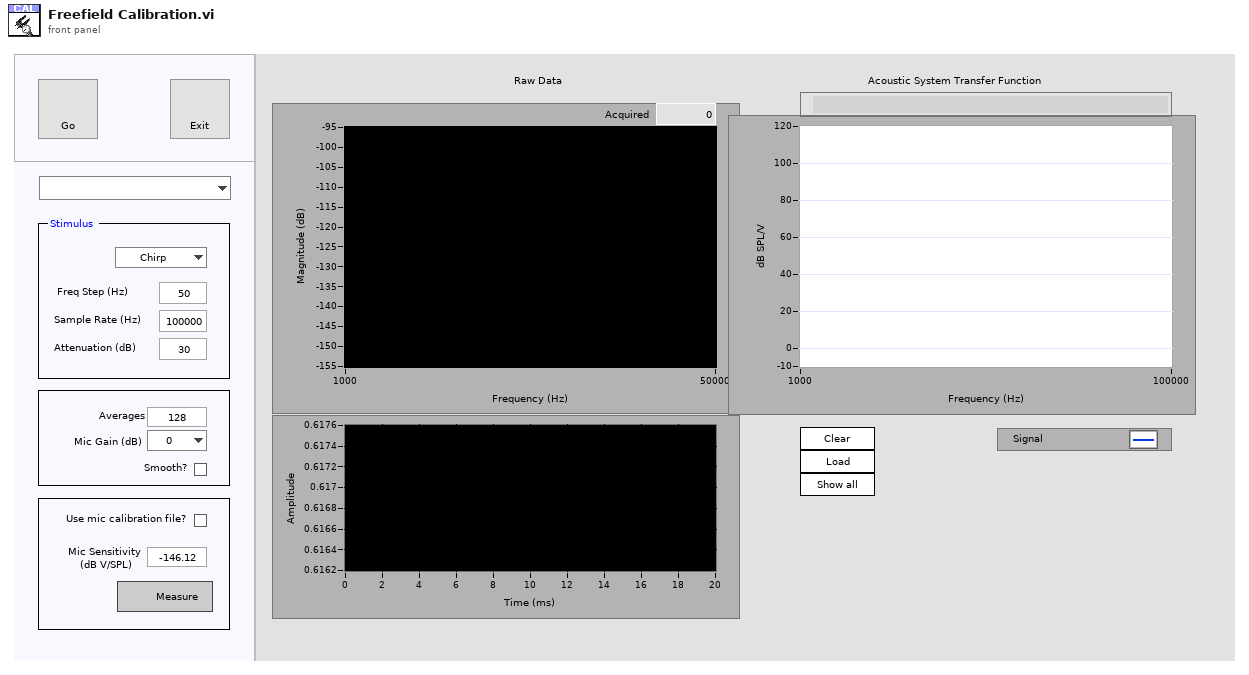
[diagram p1: front panel]
types:
  T1 = cluster{"Min Freq (Hz)":dbl, "Max Freq (Hz)":dbl, "Freq Step (Hz)":dbl, "Waveform":enum16{"Chirp"}, "Attenuation (dB)":dbl, "Sample Rate (Hz)":dbl}
  T2 = cluster{"Smooth?":bool, "Cal Mic Sens":dbl, "UseMicCal":bool, "MicCalFile ":path}
  T3 = typedef "CM-IO Type.ctl" = enum16{"Analog Outputs", "Analog Inputs", "Digital Outputs", "Digital Inputs"}
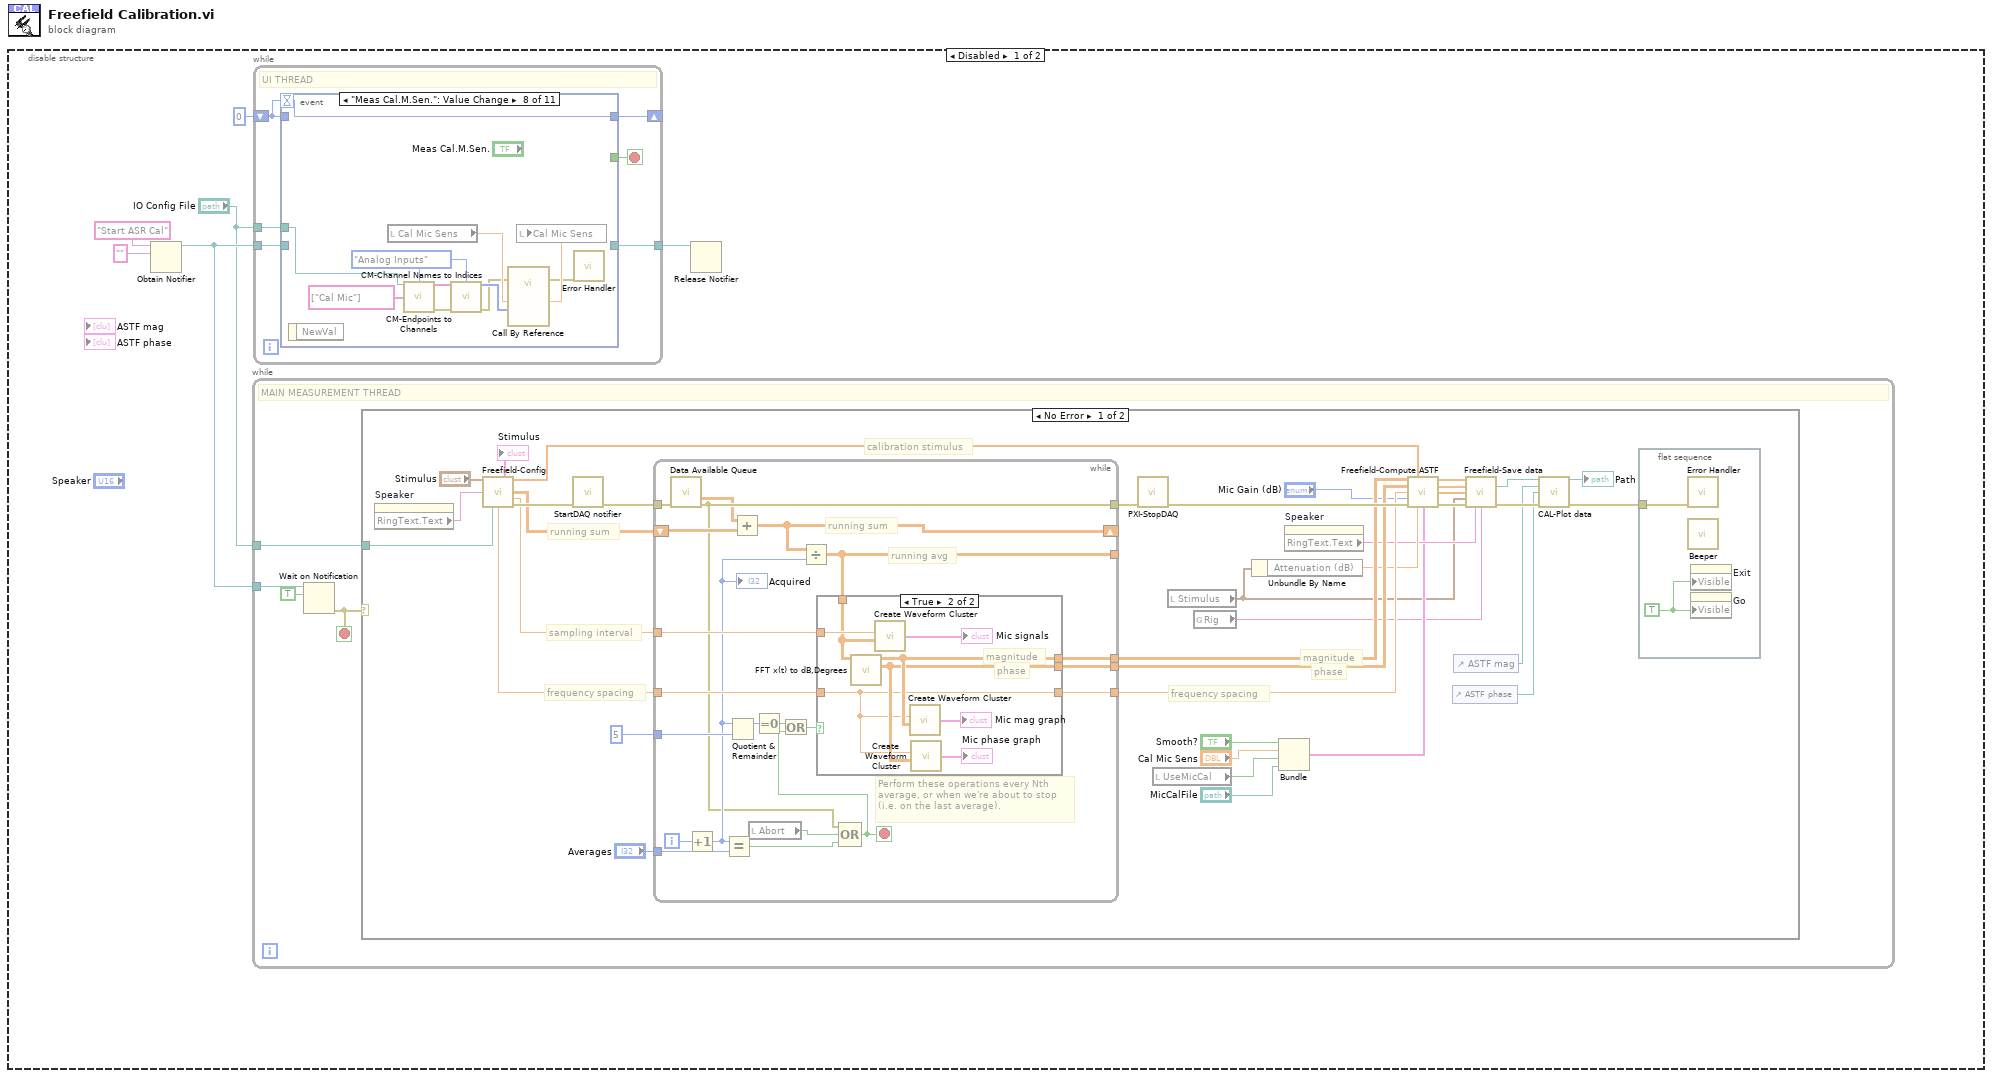
[diagram p0: block diagram]
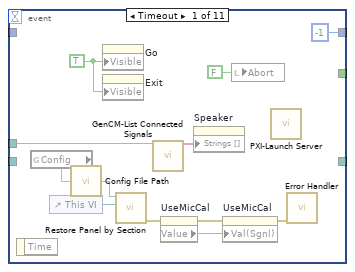
[diagram p4: hidden frame]
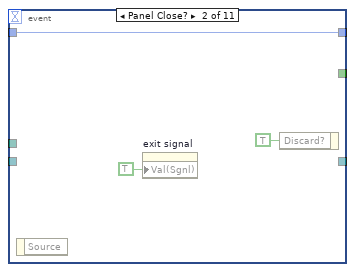
[diagram p5: hidden frame]
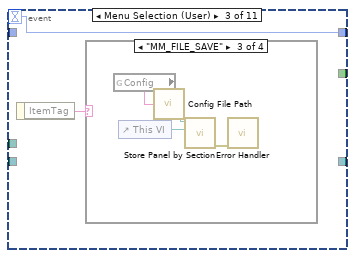
[diagram p6: hidden frame]
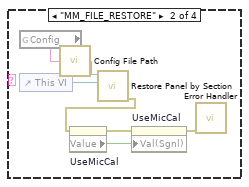
[diagram p8: hidden frame]
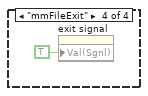
[diagram p9: hidden frame]
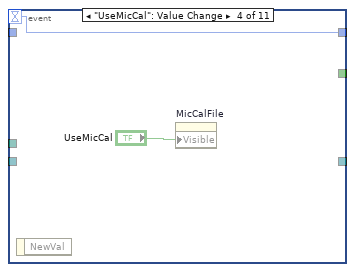
[diagram p10: hidden frame]
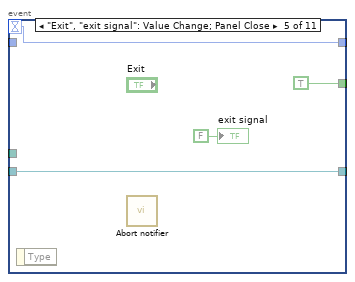
[diagram p11: hidden frame]
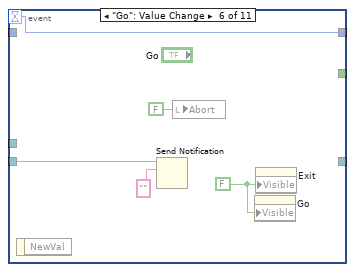
[diagram p12: hidden frame]
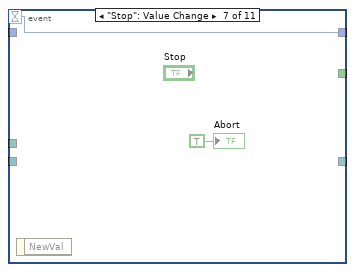
[diagram p13: hidden frame]
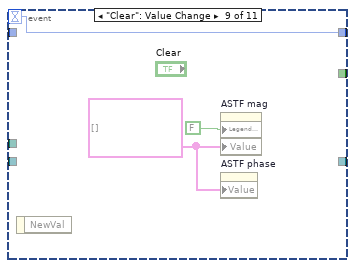
[diagram p14: hidden frame]
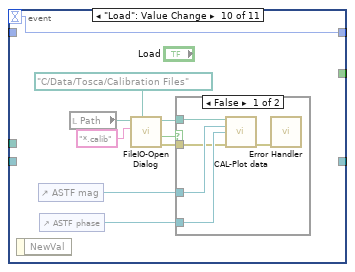
[diagram p15: hidden frame]
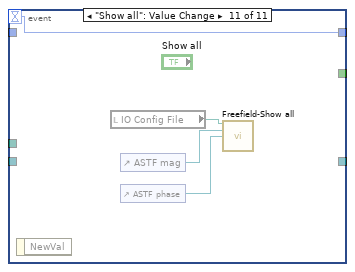
[diagram p17: hidden frame]
diagram:
  n1 = disable-structure shown="Disabled" {
    frame Disabled {
      n2 = Obtain Notifier(name (unnamed)="Start ASR Cal", notification data type="") -> (notifier out=w6:refnum<notifier>)  [unwired: 2 in, 2 out]
      n3 = while {
        tunnel: w6 -> [w9]
        tunnel: "IO Config File" -> [w7]
        stop <- w8 stop-if-true
        # "MAIN MEASUREMENT THREAD"
        n4 = Wait on Notification(notifier=w9, ignore previous (F)=TRUE) -> (error out=w8:errorcluster)  [unwired: 2 in, 3 out]
        n5 = case shown="No Error" w8 {
          tunnel: w7 -> [w13 _]
          frame No Error {
            # "phase"
            # "magnitude"
            # "frequency spacing"
            # "calibration stimulus"
            # "frequency spacing"
            # "sampling interval"
            # "running sum"
            n6 = property on="Speaker" class="Ring (strict)"() -> ("RingText.Text"=w12:string)  [unwired: 2 in, 2 out]
            n7 = call "Freefield-Config.vi"("Cal Stimulus"="Stimulus", "Speaker"=w12, "Path"=w13) -> ("Stimulus waveform"=→"Stimulus":cluster{i32, dbl, dbl[]}, "Stimulus"=w38:dbl[], "Mic Avg"=w46:dbl[][], "dt (ms)"=w44:dbl, "df (Hz)"=w45:dbl, "error out"=w47:errorcluster)  [unwired: 7 in]
            n8 = call "StartDAQ notifier.vi"("error in (no error)"=w47) -> ("error out"=w35:errorcluster)  [unwired: 6 in]
            n9 = while {
              tunnel: w35 -> [w70]
              tunnel: [w53] -> w34
              tunnel: "Averages" -> [w67]
              shift-right: [w65] -> _
              shift-left: w46 -> [w66]
              tunnel: [w51] -> _
              tunnel: 5 -> [w64]
              tunnel: w45 -> [w59]
              tunnel: [w58] -> w41
              tunnel: [w57] -> w40
              tunnel: w44 -> [w56]
              tunnel: [w55] -> w39
              i -> [w69]
              stop <- w60 stop-if-true
              # "Perform these operations every Nth\naverage, or when we're about to stop\n(i.e. on the last average)."
              # "running avg"
              # "running sum"
              n10 = call "Data Available Queue.vi"("error in (no error)"=w70) -> ("AI Waveforms"=w52:dbl[][], "error out"=w53:errorcluster)  [unwired: 10 in, 3 out]
              n11 = Increment(x=w69) -> (x+1=w54:i32)
              "Acquired" <- w54
              n12 = Equal?(x=w54, y=w67) -> (x = y?=w68:bool)
              n13 = Quotient & Remainder(x=w54, y=w64) -> (x-y*floor(x/y)=w63:i32)  [unwired: 1 out]
              n14 = Add(x=w52, y=w66) -> (x+y=w65:dbl[][])
              n15 = local read "Abort"() -> (w50:bool)
              n16 = Equal To 0?(x=w63) -> (x = 0?=w61:bool)
              n17 = Divide(x=w65, y=w54) -> (x/y=w51:dbl[][])
              n18 = Compound Arithmetic op=OR(w53, w50, w68) -> (w60:bool)
              n19 = Or(x=w61, y=w60) -> (x .or. y?=w62:bool)
              n20 = case shown="True" w62 {
                tunnel: w59 -> [_ w72]
                tunnel: [_ w76] -> w58
                tunnel: [_ w75] -> w57
                tunnel: w56 -> [_ w74]
                tunnel: [_ w72] -> w55
                tunnel: w51 -> [_ w71]
                frame False {
                }
                frame True {
                  # "phase"
                  # "magnitude"
                  n21 = call-poly "FFT x(t) to dB,Degrees.vi"("X(t)"=w71) -> ("+Freq Phase of FFT (degrees)"=w75:dbl[][], "+Freq. Mag of FFT (dB rms)"=w76:dbl[][])  [unwired: 9 in]
                  n22 = call-poly "Create Waveform Cluster.vi"("dx"=w74, "Array"=w71) -> ("waveform cluster"=→"Mic signals":cluster{"offset":dbl, "dx":dbl, "Y":dbl[][]})  [unwired: 3 in]
                  n23 = call-poly "Create Waveform Cluster.vi"("dx"=w72, "Array"=w76) -> ("waveform cluster"=→"Mic mag graph":cluster{"offset":dbl, "dx":dbl, "Y":dbl[][]})  [unwired: 3 in]
                  n24 = call-poly "Create Waveform Cluster.vi"("dx"=w72, "Array"=w75) -> ("waveform cluster"=→"Mic phase graph":cluster{"offset":dbl, "dx":dbl, "Y":dbl[][]})  [unwired: 3 in]
                }
              }
            }
            n25 = call "PXI-StopDAQ.vi"("error in (no error)"=w34) -> ("error out"=w43:errorcluster)  [unwired: 6 in]
            n26 = local read "UseMicCal"() -> (w17:bool)
            n27 = local read "Stimulus"() -> (w14:T1)
            n28 = global read "Tosca-Globals.vi" "Rig"() -> (w11:string)
            n29 = Unbundle By Name(w14) -> ("Attenuation (dB)"=w29:dbl)
            n30 = Bundle("Smooth?"="Smooth?", "Cal Mic Sens"="Cal Mic Sens", "UseMicCal"=w17, "MicCalFile"="MicCalFile") -> (w15:T2)  [unwired: 1 in]
            n31 = property on="Speaker" class="Ring (strict)"() -> ("RingText.Text"=w20:string)  [unwired: 2 in, 2 out]
            n32 = call "Freefield-Compute ASTF.vi"("Mag"=w41, "Stimulus"=w38, "Phase"=w40, "df (Hz)"=w39, "Mic Gain (dB)"="Mic Gain (dB)", "error in (no error)"=w43, "Attenuation (dB)"=w29, "Compute Options"=w15) -> ("ASTF Mag"=w30:dbl[], "ASTF Phase"=w25:dbl[], "Frequency"=w24:dbl[], "error out"=w31:errorcluster)  [unwired: 4 in]
            n33 = control-ref of="ASTF phase"() -> (w22:refnum<vi>)
            n34 = control-ref of="ASTF mag"() -> (w23:refnum<vi>)
            n35 = call "Freefield-Save data.vi"("Mag"=w30, "Phase"=w25, "Frequency"=w24, "Stimulus"=w14, "error in (no error)"=w31, "Speaker"=w20, "Rig"=w11) -> ("new file path"=w27:path, "error out"=w28:errorcluster)  [unwired: 7 in]
            n36 = call "CAL-Plot data.vi"("Path"=w27, "Mag graph"=w23, "Phase graph"=w22, "error in (no error)"=w28) -> ("Path (out)"=→"Path":path, "error out"=w42:errorcluster)  [unwired: 10 in]
            n37 = flat-sequence {
              tunnel: w42 -> [w49]
              frame #0 {
                w48 = TRUE
                n38 = call "Error Handler.vi"("error in (no error)"=w49) -> ()  [unwired: 13 in, 2 out]
                n39 = call "Beeper.vi"() -> ()  [unwired: 5 in, 1 out]
                n40 = property on="Exit" class="Bool"("Visible"=w48) -> ()  [unwired: 2 in, 2 out]
                n41 = property on="Go" class="Bool"("Visible"=w48) -> ()  [unwired: 2 in, 2 out]
              }
            }
          }
          frame Error {
          }
        }
      }
      n42 = while {
        tunnel: w6 -> [w83]
        tunnel: [w82] -> w3
        shift-right: [w81] -> _
        shift-left: 0 -> [w79]
        tunnel: "IO Config File" -> [w80]
        stop <- w84 stop-if-true
        # "UI THREAD"
        n43 = event shown="[7] \"Meas Cal.M.Sen.\": Value Change" {
          selector: _ -> [_ _ _ _ _ _ _ _ _ _ _]
          dyn-events: _ -> [_ _ _ _ _ _ _ _ _ _ _]
          timeout: w79 -> [_ _ w101 w115 w117 w121 w125 w135 w138 w147 w155]
          tunnel: [_ _ _ _ TRUE _ _ _ _ _ _] -> w84
          tunnel: w83 -> [_ _ _ _ w118 w124 _ _ _ _ _]
          tunnel: [_ _ _ _ w118 _ _ _ _ _ _] -> w82
          tunnel: [-1 w97 w101 w115 w117 w121 w125 w135 w138 w147 w155] -> w81
          tunnel: w80 -> [w86 _ _ _ _ _ _ w130 _ _ _]
          tunnel: w79 -> [_ w97 _ _ _ _ _ _ _ _ _]
          event Timeout {
            w95 = TRUE ("Visible")
            n44 = event-data() -> ()  [unwired: 1 in, 1 out]
            n45 = global read "Tosca-Globals.vi" "Config"() -> (w85:string)
            n46 = control-ref of="This VI"() -> (w91:refnum<vi>)
            n47 = call "Config File Path.vi"("AppName"=w85) -> ("Default config file name"=w90:path)
            n48 = property on="Go" class="Bool"("Visible"=w95) -> ()  [unwired: 2 in, 2 out]
            n49 = property on="Exit" class="Bool"("Visible"=w95) -> ()  [unwired: 2 in, 2 out]
            n50 = call "Restore Panel by Section.vi"("VI reference"=w91, "Path (dialog)"=w90) -> ("Error Out"=w92:errorcluster)  [unwired: 9 in]
            n51 = call "GenCM-List Connected Signals.vi"("Path"=w86) -> ("Analog Outputs"=w93:string[])  [unwired: 10 in, 4 out]
            n52 = property on="UseMicCal" class="Bool (strict)"(error in=w92) -> (error out=w89:errorcluster, "Value"=w87:bool)  [unwired: 1 in, 1 out]
            n53 = property on="Speaker" class="Ring (strict)"("Strings []"=w93) -> ()  [unwired: 2 in, 2 out]
            n54 = property on="UseMicCal" class="Bool (strict)"(error in=w89, "Val(Sgnl)"=w87) -> (error out=w88:errorcluster)  [unwired: 1 in, 1 out]
            n55 = local write "Abort"(FALSE ("Abort")) -> ()
            n56 = call "PXI-Launch Server.vi"() -> ()  [unwired: 10 in, 2 out]
            n57 = call "Error Handler.vi"("error in (no error)"=w88) -> ()  [unwired: 13 in, 2 out]
          }
          event Panel Close? {
            n58 = event-data() -> ()  [unwired: 1 in, 1 out]
            n59 = property on="exit signal" class="Bool (strict)"("Val(Sgnl)"=TRUE ("Value (Signaling)")) -> ()  [unwired: 2 in, 2 out]
            n60 = event-data("Discard?"=TRUE) -> ()  [unwired: 1 in, 1 out]
          }
          event Menu Selection (User) {
            n61 = event-data() -> ("ItemTag"=w100:string)  [unwired: 1 in]
            n62 = case shown="\"MM_FILE_SAVE\"" w100 {
              frame "False", Default {
              }
              frame "MM_FILE_RESTORE" {
                n63 = global read "Tosca-Globals.vi" "Config"() -> (w103:string)
                n64 = control-ref of="This VI"() -> (w108:refnum<vi>)
                n65 = call "Config File Path.vi"("AppName"=w103) -> ("Default config file name"=w102:path)
                n66 = call "Restore Panel by Section.vi"("VI reference"=w108, "Path (dialog)"=w102) -> ("Error Out"=w104:errorcluster)  [unwired: 9 in]
                n67 = property on="UseMicCal" class="Bool (strict)"(error in=w104) -> (error out=w105:errorcluster, "Value"=w107:bool)  [unwired: 1 in, 1 out]
                n68 = property on="UseMicCal" class="Bool (strict)"(error in=w105, "Val(Sgnl)"=w107) -> (error out=w106:errorcluster)  [unwired: 1 in, 1 out]
                n69 = call "Error Handler.vi"("error in (no error)"=w106) -> ()  [unwired: 13 in, 2 out]
              }
              frame "MM_FILE_SAVE" {
                n70 = global read "Tosca-Globals.vi" "Config"() -> (w110:string)
                n71 = control-ref of="This VI"() -> (w111:refnum<vi>)
                n72 = call "Config File Path.vi"("AppName"=w110) -> ("Default config file name"=w109:path)
                n73 = call "Store Panel by Section.vi"("VI reference"=w111, "Path (dialog)"=w109) -> ("Error Out"=w112:errorcluster)  [unwired: 9 in]
                n74 = call "Error Handler.vi"("error in (no error)"=w112) -> ()  [unwired: 13 in, 2 out]
              }
              frame "mmFileExit" {
                n75 = property on="exit signal" class="Bool (strict)"("Val(Sgnl)"=TRUE ("Value (Signaling)")) -> ()  [unwired: 2 in, 2 out]
              }
            }
          }
          event "UseMicCal": Value Change {
            n76 = event-data() -> ()  [unwired: 1 in, 1 out]
            n77 = property on="MicCalFile" class="Path"("Visible"="UseMicCal") -> ()  [unwired: 2 in, 2 out]
          }
          event "Exit", "exit signal": Value Change; Panel Close {
            n78 = event-data() -> ()  [unwired: 1 in, 1 out]
            n79 = call "Abort notifier.vi"() -> ()  [unwired: 6 in, 2 out]
            "exit signal" <- FALSE ("exit signal")
          }
          event "Go": Value Change {
            w120 = FALSE
            n80 = event-data() -> ()  [unwired: 1 in, 1 out]
            n81 = Send Notification(notification="", notifier=w124) -> ()  [unwired: 1 in, 2 out]
            n82 = local write "Abort"(FALSE ("Abort")) -> ()
            n83 = property on="Go" class="Bool"("Visible"=w120) -> ()  [unwired: 2 in, 2 out]
            n84 = property on="Exit" class="Bool"("Visible"=w120) -> ()  [unwired: 2 in, 2 out]
          }
          event "Stop": Value Change {
            n85 = event-data() -> ()  [unwired: 1 in, 1 out]
            "Abort" <- TRUE ("Abort")
          }
          event "Meas Cal.M.Sen.": Value Change {
            w132 = CM-IO_Type."Analog Inputs" ("IO Type")
            n86 = event-data() -> ()  [unwired: 1 in, 1 out]
            n87 = local read "Cal Mic Sens"() -> (w136:dbl)
            n88 = call "CM-Endpoints to Channels.vi"("Path"=w130, "IO Type"=w132, "Requested Endpoints"=string[] ["Cal Mic"] ("Inputs")) -> ("IO Channels"=w131:string[], "error out"=w133:errorcluster)  [unwired: 11 in]
            n89 = call "CM-Channel Names to Indices.vi"("IO Channels"=w131, "IO Type"=w132, "error in (no error)"=w133) -> ("Indices"=w129:i32[], "error out"=w128:errorcluster)  [unwired: 11 in]
            n90 = call-by-ref "?"(error in=w128, "AI Channels"=w129, "Mic Sens (dB V/SPL) in"=w136) -> (error out=w127:errorcluster, "Mic Sens (dB V/SPL)"=w137:dbl)  [unwired: 10 in, 1 out]
            n91 = local write "Cal Mic Sens"(w137) -> ()
            n92 = call "Error Handler.vi"("error in (no error)"=w127) -> ()  [unwired: 13 in, 2 out]
          }
          event "Clear": Value Change {
            w139 = cluster{"Frequency":dbl[], "Frequency":dbl[]}[] [] ("ASTF mag")
            n93 = event-data() -> ()  [unwired: 1 in, 1 out]
            n94 = property on="ASTF mag" class="XYGraph (strict)"("Legend Visible"=FALSE ("Legend:Visible"), "Value"=w139) -> ()  [unwired: 2 in, 2 out]
            n95 = property on="ASTF phase" class="XYGraph (strict)"("Value"=w139) -> ()  [unwired: 2 in, 2 out]
          }
          event "Load": Value Change {
            n96 = event-data() -> ()  [unwired: 1 in, 1 out]
            n97 = control-ref of="ASTF mag"() -> (w149:refnum<vi>)
            n98 = control-ref of="ASTF phase"() -> (w148:refnum<vi>)
            n99 = local read "Path"() -> (w143:path)
            n100 = call "FileIO-Open Dialog.vi"("Default Folder"=path "C:/Data/Tosca/Calibration Files", "pattern (all files)"="*.calib", "Start path"=w143) -> ("error out"=w146:errorcluster, "cancelled"=w145:bool, "selected path"=w144:path)  [unwired: 6 in]
            n101 = case shown="False" w145 {
              tunnel: w144 -> [w154 _]
              tunnel: w149 -> [w153 _]
              tunnel: w148 -> [w152 _]
              tunnel: w146 -> [w150 _]
              frame False {
                n102 = call "CAL-Plot data.vi"("Path"=w154, "Mag graph"=w153, "Phase graph"=w152, "error in (no error)"=w150) -> ("error out"=w151:errorcluster)  [unwired: 10 in, 1 out]
                n103 = call "Error Handler.vi"("error in (no error)"=w151) -> ()  [unwired: 13 in, 2 out]
              }
              frame True {
              }
            }
          }
          event "Show all": Value Change {
            n104 = event-data() -> ()  [unwired: 1 in, 1 out]
            n105 = local read "IO Config File"() -> (w156:path)
            n106 = control-ref of="ASTF mag"() -> (w158:refnum<vi>)
            n107 = control-ref of="ASTF phase"() -> (w157:refnum<vi>)
            n108 = call "Freefield-Show all.vi"("Path"=w156, "Mag graph"=w158, "Phase graph"=w157) -> ()  [unwired: 12 in, 1 out]
          }
        }
      }
      n109 = Release Notifier(notifier=w3) -> ()  [unwired: 2 in, 3 out]
    }
    frame Enabled {
    }
  }
